vi "arm set point.vi"(1 "Setpoint In":dbl format="%#_13g", 2 "Menu":T1) -> (0 "Setpoint Out":dbl)   [LabVIEW 2013]
uses:
  typedefs/fg_typedef.ctl
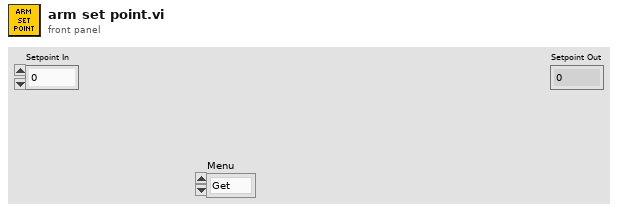
[diagram p1: front panel]
types:
  T1 = typedef "fg_typedef.ctl" = enum16{"Get", "Set"}
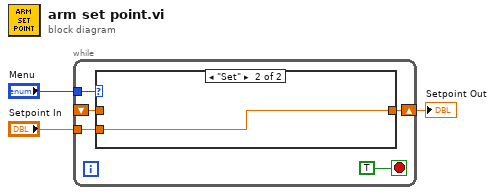
[diagram p0: block diagram]
diagram:
  n1 = while {
    tunnel: "Menu" -> [w7]
    tunnel: "Setpoint In" -> [w6]
    shift-right: [w5] -> w1
    shift-left: _ -> [w4]
    stop <- TRUE stop-if-true
    n2 = case shown="\"Set\"" w7 {
      tunnel: w6 -> [_ w10]
      tunnel: [w9 w10] -> w5
      tunnel: w4 -> [w9 _]
      frame "Get", Default {
      }
      frame "Set" {
      }
    }
  }
  "Setpoint Out" <- w1
